vi "Send Done.vi"(7 "Message Priority (Normal)":T1=enum."Normal", 8 "error in (no error)":errorcluster, 10 "Philosopher ID":i32, 11 "Table:Done Eating Msg":refnum<class "Message Enqueuer.lvclass">) -> (0 "error out":errorcluster, 3 "Table:Done Eating Msg":refnum<class "Message Enqueuer.lvclass">)   [LabVIEW 2023, in "Table.lvlib" / "Done Eating.lvclass"]
doc: "This VI sends the message to an actor."
uses:
  Done Eating.lvclass
  <vilib>/ActorFramework/Message Enqueuer/Message Enqueuer.lvclass
  <vilib>/ActorFramework/Message Enqueuer/Message Priority.ctl
  C:/Program Files (x86)/National Instruments/LabVIEW 2023/vi.lib/ActorFramework/Message/Message.lvclass
  Done Eating.lvclass/Done Eating.ctl
  <vilib>/ActorFramework/Message Enqueuer/Message Enqueuer.lvclass/Message Enqueuer.ctl
  <vilib>/ActorFramework/Message Priority Queue/Priority Enqueue.vi
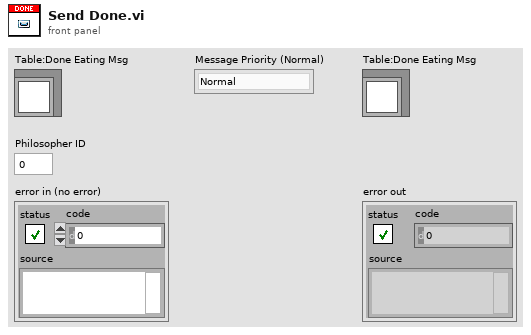
[diagram p1: front panel]
types:
  T1 = typedef "Actor Framework.lvlib/Message Enqueuer.lvclass/Message Priority.ctl" = enum16{"Low", "Normal", "High"}
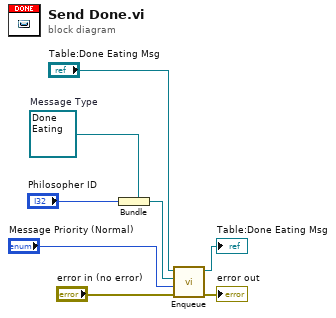
[diagram p0: block diagram]
diagram:
  w5 = refnum<class "Done Eating.lvclass"> refnum  # Message Type
  n1 = Bundle(cluster=w5, "Philosopher ID") -> (w4:refnum<class "Done Eating.lvclass">)
  n2 = call <vilib>:"Enqueue.vi"("error in (no error)"="error in (no error)", "Message Priority (Normal)"="Message Priority (Normal)", "Message"=w4, "Message Enqueuer in"="Table:Done Eating Msg") -> ("error out"=→"error out":errorcluster, "Message Enqueuer out"=→"Table:Done Eating Msg":refnum<class "Message Enqueuer.lvclass">)  [unwired: 6 in]
